vi "MainPreview.vi"(8 "Error":errorcluster) -> (0 "Error Out":errorcluster, 3 "Elements In Queue Out":T1[](array[typedef]))   [LabVIEW 2022 SP3]
doc: "The function reads the elements in the queue but does not remove them. This can be used in storing data in the queue and retrieving from multiple locations."
uses:
  Type Def/MainStates Cluster.ctl
  Type Def/MainStates.ctl
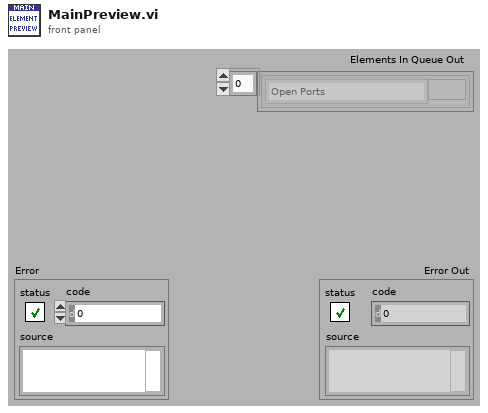
[diagram p1: front panel]
types:
  T1 = typedef "MainStates Cluster.ctl" = cluster{"States":T2, "Data":variant}
  T2 = typedef "MainStates.ctl" = enum16{"Open Ports", "Close Ports", "Main", "Settings", "Voltaje", "Probe", "Lenguaje", "Callibration", "Exit", "Voltage Test", "Test 2", "End test"}
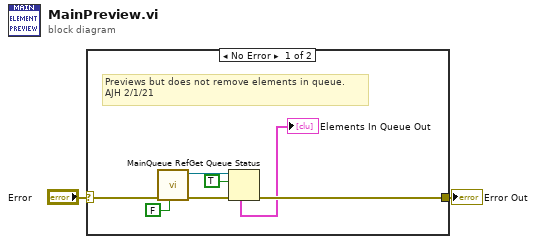
[diagram p0: block diagram]
diagram:
  n1 = case shown="No Error" "Error" {
    selector: "Error" -> [w8 w10]
    tunnel: [w6 w10] -> w1
    frame No Error {
      # "Previews but does not remove elements in queue.\nAJH 2/1/21"
      n2 = call "MainQueue Ref.vi"("Write:T/Read:(F)"=FALSE ("Write:T/Read:F"), "error in"=w8) -> ("error out"=w7:errorcluster, "queue out"=w5:refnum<queue>)  [unwired: 8 in]
      n3 = Get Queue Status(queue=w5, return elements? (F)=TRUE, error in (no error)=w7) -> (error out=w6:errorcluster, elements=→"Elements In Queue Out":T1[])  [unwired: 6 out]
    }
    frame Error {
    }
  }
  "Error Out" <- w1
